vi "Config_Execute_Write_TSP.vi"(0 "VISA Refnum in":refnum<visa-resource-name>, 1 "Saved Folder:":path, 2 "Ambient Temp (Y/N)":bool, 3 "SMU4? (Y/N)":bool, 5 "TSP Cluster":T6, 7 "SMU Config":T1={"Vname"="Vs", "Vname 2"="Vd", "Vname 3"="Vg", "Vname 4"="V4", "Iname"="Is", "Iname 2"="Id", "Iname 3"="Ig", "Iname 4"="I4", "Mode"=4, "Mode 2"=0, "Mode 3"=0, "Mode 4"=0, "Function"=4, "Function 2"=1, "Function 3"=2, "Function 4"=4, "Value (V or A)"=0.0, "Value (Either V or A) 2"=0.0, "Value (Either V or A) 3"=0.0, "Value (Either V or A) 4"=0.0} {"Function" items=["disabled", "Var1", "Var2", "Var1'", "Constant"]; "Mode" items=["V", "I", "VPulse", "IPulse", "Common"]; "Function 4" items=["disabled", "Var1", "Var2", "Var1'", "Constant"]; "Mode 4" items=["V", "I", "VPulse", "IPulse", "Common"]; "Function 3" items=["disabled", "Var1", "Var2", "Var1'", "Constant"]; "Mode 3" items=["V", "I", "VPulse", "IPulse", "Common"]; "Function 2" items=["disabled", "Var1", "Var2", "Var1'", "Constant"]; "Mode 2" items=["V", "I", "VPulse", "IPulse", "Common"]}, 9 "Graph Cluster in":T3, 10 "Sample Properties:":T5, 11 "error In":errorcluster, 12 "Gate Current Cluster":T4, 14 "Compliance Cluster":T2) -> (4 "Filepath Out":path, 6 "Graph Cluster out":T3, 15 "error Out":errorcluster)   [LabVIEW 2012]
panel:
  # "SMU1"
  # "SMU2"
  # "SMU3"
  # "SMU4"
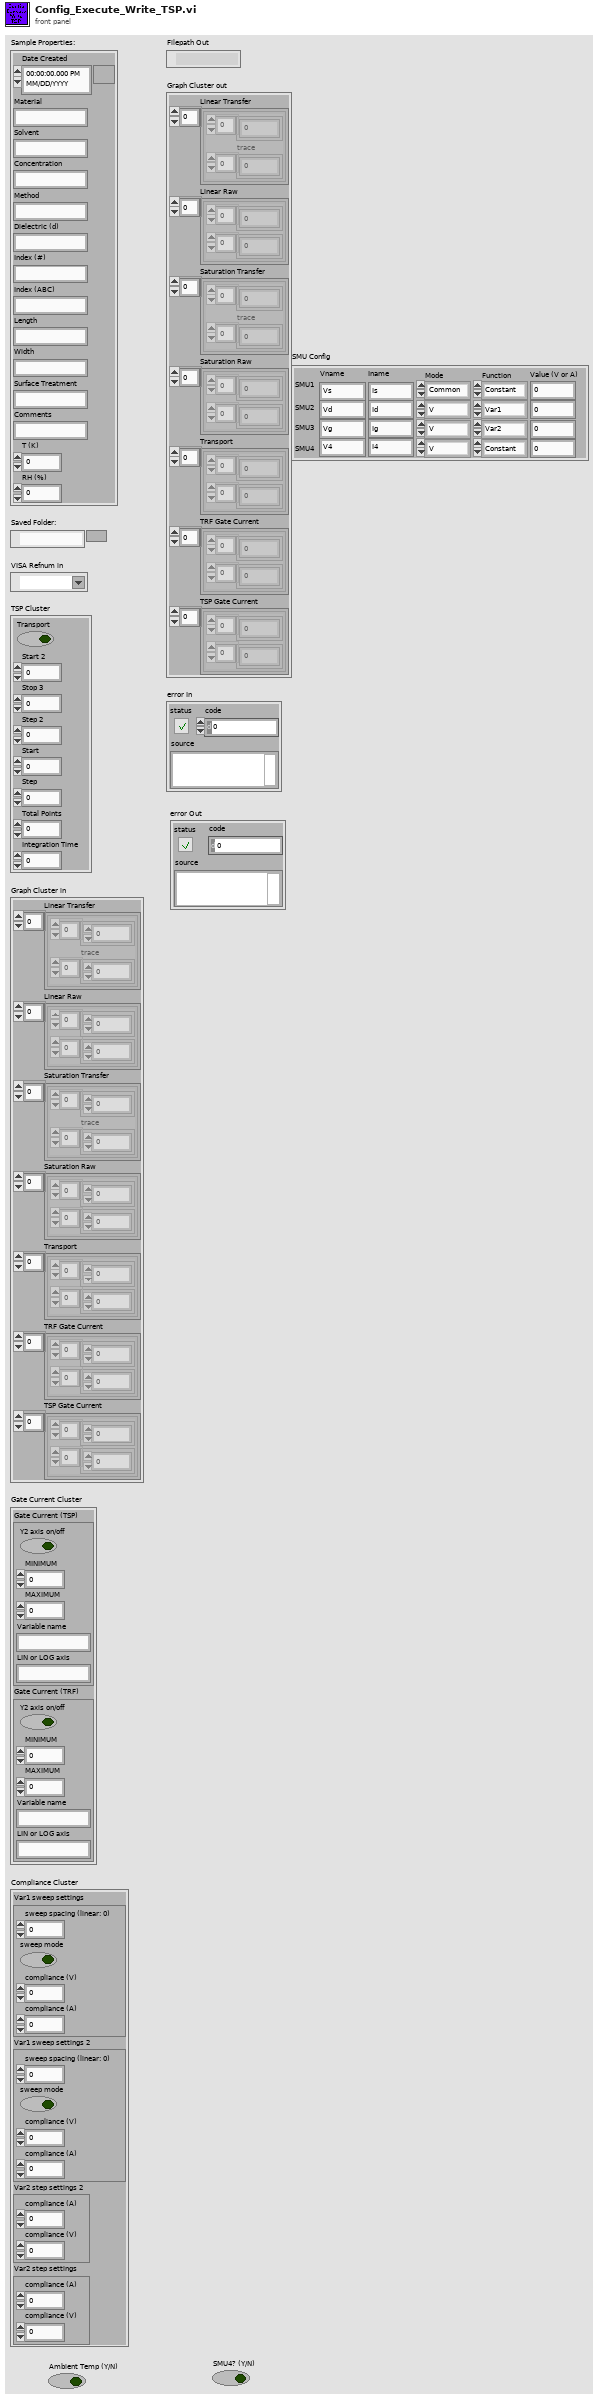
[diagram p1: front panel]
types:
  T1 = cluster{"Vname":string, "Vname 2":string, "Vname 3":string, "Vname 4":string, "Iname":string, "Iname 2":string, "Iname 3":string, "Iname 4":string, "Mode":u16, "Mode 2":u16, "Mode 3":u16, "Mode 4":u16, "Function":u16, "Function 2":u16, "Function 3":u16, "Function 4":u16, "Value (V or A)":dbl, "Value (Either V or A) 2":dbl, "Value (Either V or A) 3":dbl, "Value (Either V or A) 4":dbl}
  T2 = cluster{"Var1 sweep settings":cluster{"sweep spacing (linear: 0)":u16, "sweep mode":bool, "compliance (V)":dbl, "compliance (A)":dbl}, "Var1 sweep settings 2":cluster{"sweep spacing (linear: 0)":u16, "sweep mode":bool, "compliance (V)":dbl, "compliance (A)":dbl}, "Var2 step settings 2":cluster{"compliance (A)":dbl, "compliance (V)":dbl}, "Var2 step settings":cluster{"compliance (A)":dbl, "compliance (V)":dbl}}
  T3 = cluster{"Linear Transfer":cluster{dbl[], "trace":dbl[]}[], "Linear Raw":cluster{dbl[], dbl[]}[], "Saturation Transfer":cluster{dbl[], "trace":dbl[]}[], "Saturation Raw":cluster{dbl[], dbl[]}[], "Transport":cluster{dbl[], dbl[]}[], "TRF Gate Current":cluster{dbl[], dbl[]}[], "TSP Gate Current":cluster{dbl[], dbl[]}[]}
  T4 = cluster{"Gate Current (TSP)":cluster{"Y2 axis on/off":bool, "MINIMUM":ext, "MAXIMUM":ext, "Variable name":string, "LIN or LOG axis":string}, "Gate Current (TRF)":cluster{"Y2 axis on/off":bool, "MINIMUM":ext, "MAXIMUM":ext, "Variable name":string, "LIN or LOG axis":string}}
  T5 = cluster{"Date Created":timestamp, "Material":string, "Solvent":string, "Concentration":string, "Method":string, "Dielectric (d)":string, "Index (#)":string, "Index (ABC)":string, "Length":string, "Width":string, "Surface Treatment":string, "Comments":string, "T (K)":dbl, "RH (%)":dbl}
  T6 = cluster{"Transport":bool, "Start 2":dbl, "Stop 3":dbl, "Step 2":dbl, "Start":dbl, "Step":dbl, "Total Points":u16, "Integration Time":u32}
  T7 = cluster{"sweep spacing (linear: 0)":u16, "sweep mode":bool, "compliance (V)":dbl, "compliance (A)":dbl}
  T8 = cluster{"compliance (A)":dbl, "compliance (V)":dbl}
  T9 = cluster{"Y2 axis on/off":bool, "MINIMUM":ext, "MAXIMUM":ext, "Variable name":string, "LIN or LOG axis":string}
  T10 = cluster{"Start 2":dbl, "Stop 3":dbl, "Step 2":dbl, "sweep spacing (linear: 0)":u16, "sweep mode":bool, "compliance (V)":dbl, "compliance (A)":dbl}
  T11 = cluster{"compliance (A)":dbl, "compliance (V)":dbl, "Start":dbl, "Total Points":u16, "Step":dbl}
  T12 = cluster{"Transport":cluster{dbl[], dbl[]}[], "Gate Current":cluster{dbl[], dbl[]}[]}
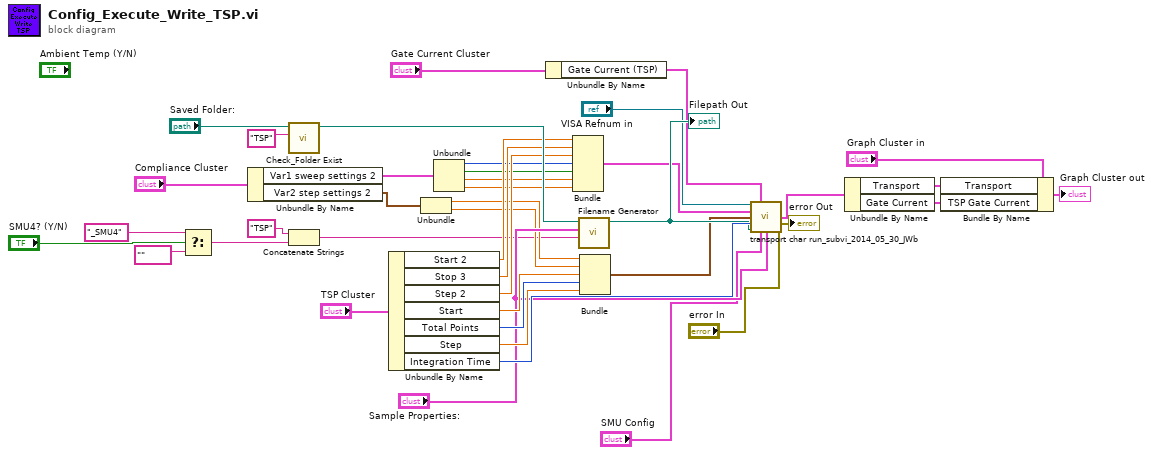
[diagram p0: block diagram]
diagram:
  n1 = Select(t="_SMU4", s="SMU4? (Y/N)", f="") -> (s? t:f=w7:string)
  n2 = Unbundle By Name("Compliance Cluster") -> ("Var1 sweep settings 2"=w23:T7, "Var2 step settings 2"=w24:T8)
  n3 = call "Check_Folder Exist.vi"("Folder Name"="TSP", "Root Folder"="Saved Folder:") -> ("Output Path"=w34:path)  [unwired: 9 in]
  n4 = Concatenate Strings("TSP", w7) -> (w2:string)
  n5 = Unbundle By Name("TSP Cluster") -> ("Start 2"=w18:dbl, "Stop 3"=w19:dbl, "Step 2"=w20:dbl, "Start"=w40:dbl, "Total Points"=w39:u16, "Step"=w38:dbl, "Integration Time"=w41:u32)
  n6 = Unbundle(w24) -> ("compliance (A)"=w15:dbl, "compliance (V)"=w16:dbl)
  n7 = Unbundle(w23) -> ("sweep spacing (linear: 0)"=w10:u16, "sweep mode"=w11:bool, "compliance (V)"=w12:dbl, "compliance (A)"=w13:dbl)
  n8 = Unbundle By Name("Gate Current Cluster") -> ("Gate Current (TSP)"=w31:T9)
  n9 = Bundle("Start 2"=w18, "Stop 3"=w19, "Step 2"=w20, "sweep spacing (linear: 0)"=w10, "sweep mode"=w11, "compliance (V)"=w12, "compliance (A)"=w13) -> (w14:T10)  [unwired: 1 in]
  n10 = call "Filename Generator.vi"("Measurement Type"=w2, "Sample Properties:"="Sample Properties:", "Saved Folder:"=w34) -> ("Filepath Out"=w36:path)  [unwired: 8 in]
  "Filepath Out" <- w36
  n11 = Bundle("compliance (A)"=w15, "compliance (V)"=w16, "Start"=w40, "Total Points"=w39, "Step"=w38) -> (w1:T11)  [unwired: 1 in]
  n12 = call "transport char run_subvi_2014_05_30_JWb.vi"("VISA session"="VISA Refnum in", "Y2 axis settings"=w31, "Var1 sweep settings"=w14, "Var2 step settings"=w1, "integration time"=w41, "Path"=w36, "SMU Config"="SMU Config", "Sample Properties:"="Sample Properties:", "error?"="error In") -> ("Graph Cluster"=w25:T12, "Error Out"=→"error Out":errorcluster)  [unwired: 4 in, 1 out]
  n13 = Unbundle By Name(w25) -> ("Transport"=w28:cluster{dbl[], dbl[]}[], "Gate Current"=w29:cluster{dbl[], dbl[]}[])
  n14 = Bundle By Name(cluster="Graph Cluster in", "Transport"=w28, "TSP Gate Current"=w29) -> (→"Graph Cluster out":T3)
